vi "PCO_GetColorCorrectionMatrix.vi"(8 "error in (no error)":errorcluster {"code" format="%x"}, 11 "ph":u64) -> (0 "error out":errorcluster {"code" format="%x"}, 1 "pdMatrix":dbl[](array[numeric]), 2 "ErrorMessage":i32 format="%x", 3 "ph out":u64)   [LabVIEW 2020, in "SDK.lvlib" / "GeneralCameraStatus.lvlib"]
doc: "<b>Description:</b>\nThis function returns the color multiplier matrix from the camera. The color multiplier matrix can be used to normalize the color values of a color camera to a color temperature of 6500k.\nThe color multiplier matrix is specific for each camera and is determined through a special calibration procedure.\n\n<b>Supported camera type:</b>\npco.dimax, pco.edge, pco.pixelfly usb\n\n<b>Descriptor dependency:</b>\ndwGeneralCapsDESC1: CCM"
uses:
  GeneralCameraStatus.lvlib
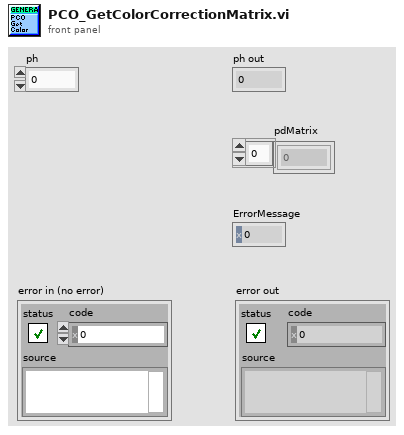
[diagram p1: front panel]
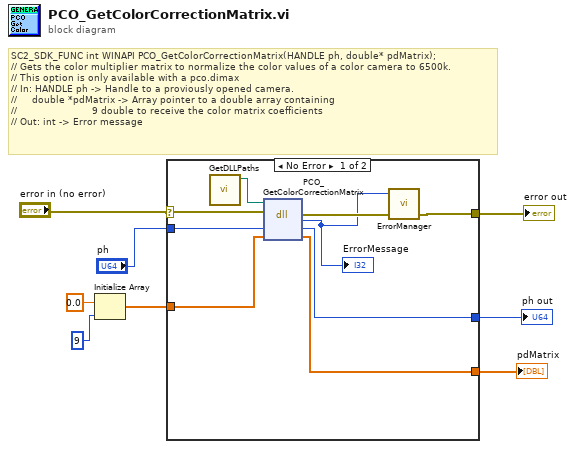
[diagram p0: block diagram]
diagram:
  # "SC2_SDK_FUNC int WINAPI PCO_GetColorCorrectionMatrix(HANDLE ph, double* pdMatrix);\n// Gets the color multiplier matrix to normalize the color values of a color camera to 6500k.\n// This option is only available with a pco.dimax\n// In: HANDLE ph -> Handle to a proviously opened camera.\n//     double *pdMatrix -> Array pointer to a double array containing\n//                         9 double to receive the color matrix coefficients\n// Out: int -> Error message"
  n1 = Initialize Array(0.0 ("element"), 9 ("dimension size")) -> (w1:dbl[])
  n2 = case shown="No Error" "error in (no error)" {
    selector: "error in (no error)" -> [w14 w19]
    tunnel: [w16 w19] -> w8
    tunnel: "ph" -> [w17 w20]
    tunnel: [w12 w18] -> w5
    tunnel: [w11 w20] -> w4
    tunnel: w1 -> [w10 w18]
    frame No Error {
      n3 = call "GetDLLPaths.vi"() -> ("SC2_Cam_Path"=w9:path)  [unwired: 9 in, 2 out]
      n4 = dll-call lib="?" fn="PCO_GetColorCorrectionMatrix"(path in=w9, error in=w14, "ph"=w17, "pdMatrix"=w10) -> (error out=w15:errorcluster, "return type"=w13:i32, "ph"=w11:u64, "pdMatrix"=w12:dbl[])  [unwired: 1 in, 1 out]
      "ErrorMessage" <- w13
      n5 = call "ErrorManager.vi"("error in (no error)"=w15, "error code"=w13) -> ("error out"=w16:errorcluster)  [unwired: 3 in]
    }
    frame Error {
    }
  }
  "error out" <- w8
  "pdMatrix" <- w5
  "ph out" <- w4
